vi "Read Macro Steps.vi"(8 "error in (no error)":errorcluster, 10 "Schema Version":string, 11 "refnum":T5) -> (0 "error out":errorcluster, 2 "Macro Steps":T1[](array[typedef]), 3 "refnum out":T5)   [LabVIEW 2020, in "MacroAssert.lvlib"]
doc: "Reads the list of steps from macro config file defined by <B>refnum</B>."
uses:
  MacroAssert.lvlib
  <vilib>/Utility/config.llb/NI_LVConfig.lvlib
  CTLs/Step Type V3.ctl
  CTLs/Step V3.ctl
  <vilib>/ErrorRing/Error Ring.xnode
  <vilib>/Utility/config.llb/Read Key (String).vi
  <vilib>/Utility/config.llb/Read Key (I32).vi
  CTLs/Assertion Type.ctl
  <vilib>/Utility/error.llb/Error Cluster From Error Code.vi
  <vilib>/picture/picture.llb/imagedata.ctl
  <vilib>/Utility/config.llb/Config Data RefNum.ctl
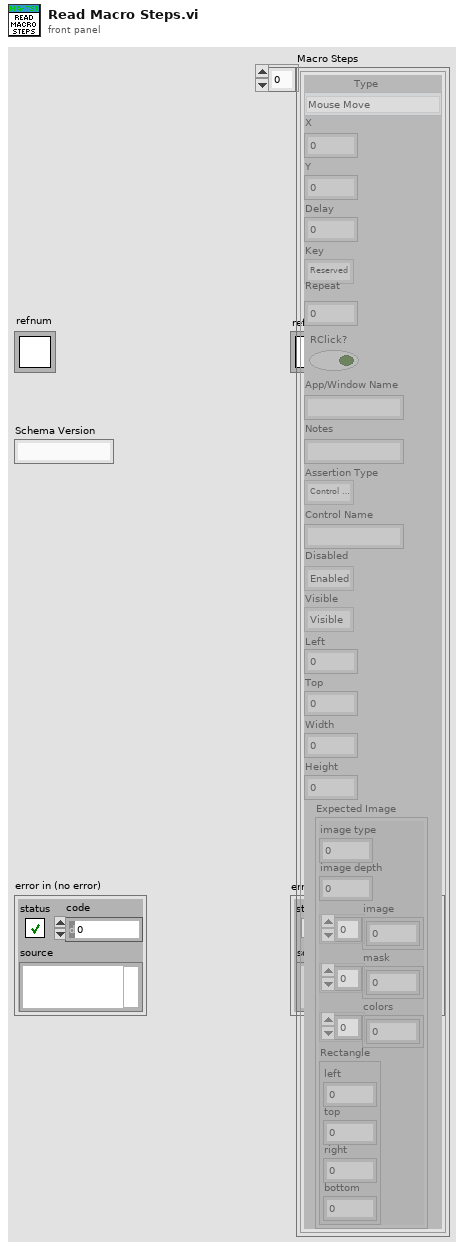
[diagram p1: front panel]
types:
  T1 = typedef "MacroAssert.lvlib/Step V3.ctl" = cluster{"Type":T2, "X":i32, "Y":i32, "Delay":i32, "Key":u8, "Repeat":i32, "RClick?":bool, "App/Window Name":string, "Notes":string, "Assertion Type":T3, "Control Name":string, "Disabled":enum8{"Enabled", "Disabled", "Disabled and Grayed Out"}, "Visible":enum16{"Visible", "Not Visible"}, "Left":i16, "Top":i16, "Width":i16, "Height":i16, "Expected Image":T4}
  T2 = typedef "MacroAssert.lvlib/Step Type V3.ctl" = enum16{"Mouse Move", "Mouse Click", "Key Press", "Wait", "Mouse Down", "Mouse Up", "Key Down", "Key Up", "Test Assertion", "Run Application", "Maximize Window", "Restore Window", "Minimize Window", "Close Window", "Bring Window to Front", "Send Window to Back"}
  T3 = typedef "MacroAssert.lvlib/Assertion Type.ctl" = enum16{"Control Position", "Control Visible", "Control Disabled", "Control Image"}
  T4 = typedef "imagedata.ctl" = cluster{"image type":i32, "image depth":i32, "image":u8[], "mask":u8[], "colors":u32[], "Rectangle":cluster{"left":i16, "top":i16, "right":i16, "bottom":i16}}
  T5 = typedef "NI_LVConfig.lvlib/Config Data RefNum.ctl" = refnum<k1>
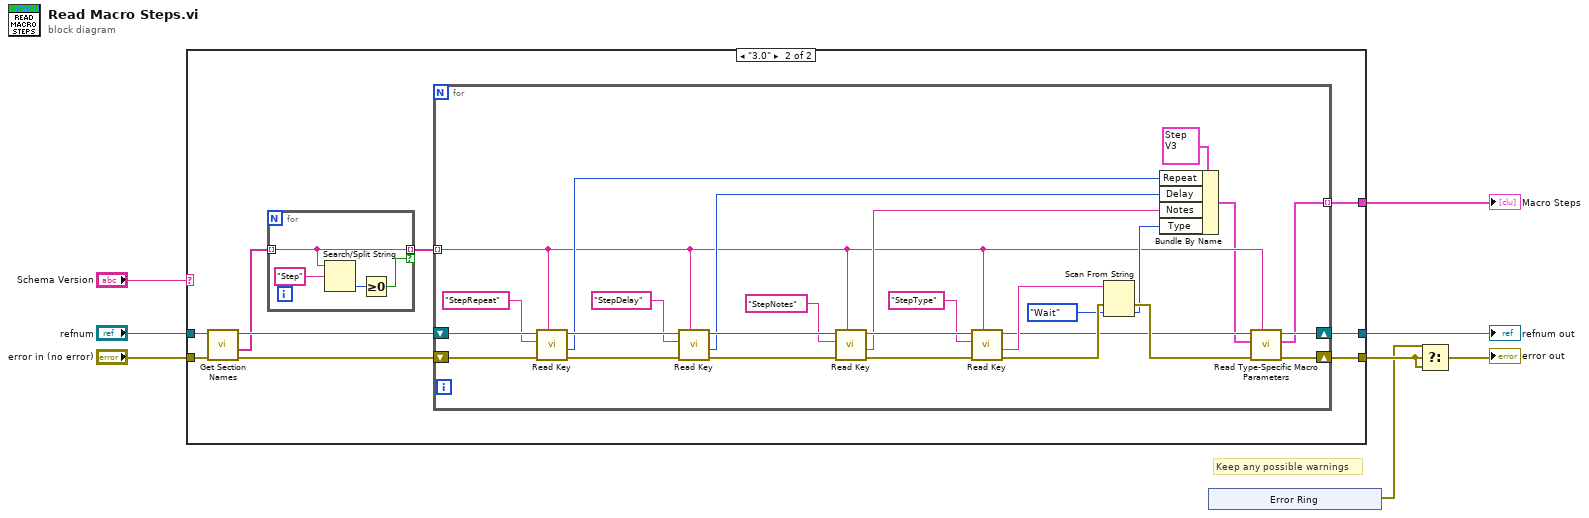
[diagram p0: block diagram]
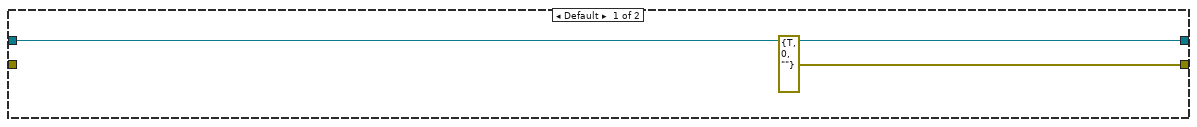
[diagram p2: hidden frame]
diagram:
  # "Keep any possible warnings"
  n1 = case shown="\"3.0\"" "Schema Version" {
    tunnel: "refnum" -> [w10 w16]
    tunnel: [w10 w18] -> w2
    tunnel: [errorcluster {"status"=TRUE, "code"=0, "source"=""} ("error out") w19] -> w8
    tunnel: "error in (no error)" -> [_ w17]
    tunnel: [_ w12] -> w1
    frame Default {
    }
    frame "3.0" {
      n2 = call <vilib>:"Get Section Names.vi"("error in (no error)"=w17, "refnum"=w16) -> ("error out"=w15:errorcluster, "section names"=w13:string[], "refnum out"=w14:T5)  [unwired: 7 in]
      n3 = for {
        tunnel: w13 -> [w47] mode=indexing
        tunnel: [w47] -> w11 mode=indexing if=w48
        n4 = Search/Split String(string=w47, search string/char (-)="Step") -> (offset of match=w49:i32)  [unwired: 1 in, 2 out]
        n5 = Greater Or Equal To 0?(x=w49) -> (x >= 0?=w48:bool)
      }
      n6 = for {
        tunnel: [w20] -> w12 mode=indexing
        shift-right: [w25] -> w19
        shift-left: w15 -> [w40]
        shift-right: [w22] -> w18
        shift-left: w14 -> [w41]
        tunnel: w11 -> [w24] mode=indexing
        n7 = call-poly <vilib>:"Read Key.vi"("section"=w24, "error in (no error)"=w40, "key"="StepRepeat", "refnum"=w41) -> ("error out"=w35:errorcluster, "value"=w29:i32, "refnum out"=w42:T5)  [unwired: 4 in, 1 out]
        n8 = call-poly <vilib>:"Read Key.vi"("section"=w24, "error in (no error)"=w35, "key"="StepDelay", "refnum"=w42) -> ("error out"=w34:errorcluster, "value"=w28:i32, "refnum out"=w44:T5)  [unwired: 4 in, 1 out]
        n9 = call-poly <vilib>:"Read Key.vi"("section"=w24, "error in (no error)"=w34, "key"="StepNotes" ("section"), "refnum"=w44) -> ("error out"=w32:errorcluster, "value"=w27:string, "refnum out"=w43:T5)  [unwired: 4 in, 1 out]
        n10 = call-poly <vilib>:"Read Key.vi"("section"=w24, "error in (no error)"=w32, "key"="StepType", "refnum"=w43) -> ("error out"=w45:errorcluster, "value"=w33:string, "refnum out"=w23:T5)  [unwired: 4 in, 1 out]
        n11 = Scan From String(input string=w33, error in=w45, default 1=Step_Type_V3."Wait" ("Step Type")) -> (error out=w46:errorcluster, output 1=w26:T2)  [unwired: 2 in, 2 out]
        n12 = Bundle By Name(cluster=T1 {"Type"=enum."Mouse Move", "X"=0, "Y"=0, "Delay"=0, "Key"=65, "Repeat"=0, "RClick?"=FALSE, "App/Window Name"="", "Notes"="", "Assertion Type"=enum."Control Position", "Control Name"="", "Disabled"=enum."Enabled", "Visible"=enum."Visible", "Left"=0, "Top"=0, "Width"=0, "Height"=0, "Expected Image"={"image type"=0, "image depth"=0, "image"=[], "mask"=[], "colors"=[], "Rectangle"={"left"=0, "top"=0, "right"=0, "bottom"=0}}} ("Step"), "Repeat"=w29, "Delay"=w28, "Notes"=w27, "Type"=w26) -> (w21:T1)
        n13 = call "Read Type-Specific Macro Parameters.vi"("Section"=w24, "error in (no error)"=w46, "Macro Step"=w21, "refnum"=w23) -> ("error out"=w25:errorcluster, "Macro Step out"=w20:T1, "refnum out"=w22:T5)  [unwired: 5 in]
      }
    }
  }
  "refnum out" <- w2
  "Macro Steps" <- w1
  n14 = xnode "Error Ring"() -> ("error out"=w7:errorcluster)
  n15 = Select(t=w7, s=w8, f=w8) -> (s? t:f=→"error out":errorcluster)
